vi "Acquisition Message Loop.vi"(6 "List Notifier":refnum<notifier>, 8 "error in (no error)":errorcluster, 9 "Data Queue":refnum<queue>, 10 "Data Notifier":refnum<notifier>, 11 "Message Queues":T1) -> (0 "error out":errorcluster)   [LabVIEW 2022 SP3, in "Acquisition.lvlib"]
doc: "Message loop for handling messages pertaining to the acquisition of data from the hardware."
uses:
  Acquisition.lvlib
  support/Message Queue/All Message Queues.ctl
  support/Message Queue/Message Cluster.ctl
  Hardware Configuration.ctl
  Acquisition State.ctl
  support/Message Queue/Enqueue Message (Single).vi
  <vilib>/Utility/error.llb/Error Cluster From Error Code.vi
  <vilib>/ErrorRing/Error Ring.xnode
  support/Message Queue/Message Queue.lvlib
  <instrlib>/BK Precision 911X Series/BK Precision 911X Series.lvlib
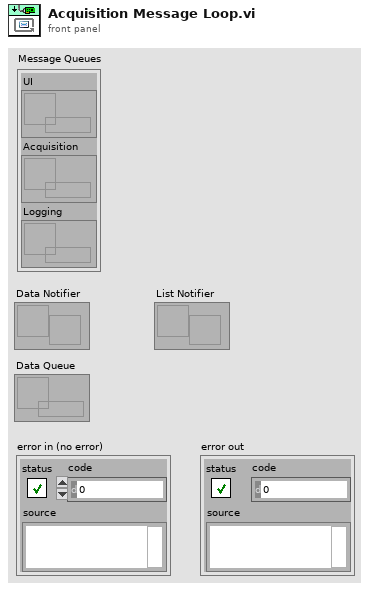
[diagram p1: front panel]
types:
  T1 = typedef "Message Queue.lvlib/All Message Queues.ctl" = cluster{"UI":refnum<queue>, "Acquisition":refnum<queue>, "Logging":refnum<queue>}
  T2 = typedef "Acquisition.lvlib/Hardware Configuration.ctl" = cluster{"VISA resource name":refnum<visa-resource-name>, "Baud Rate":u32, "Reset on Connect":bool, "Log Interval (s)":dbl, "Voltage":refnum<vi>, "Current":refnum<vi>, "Output Control":refnum<vi>}
  T3 = typedef "Acquisition.lvlib/Acquisition State.ctl" = enum16{"Idle", "Acquiring"}
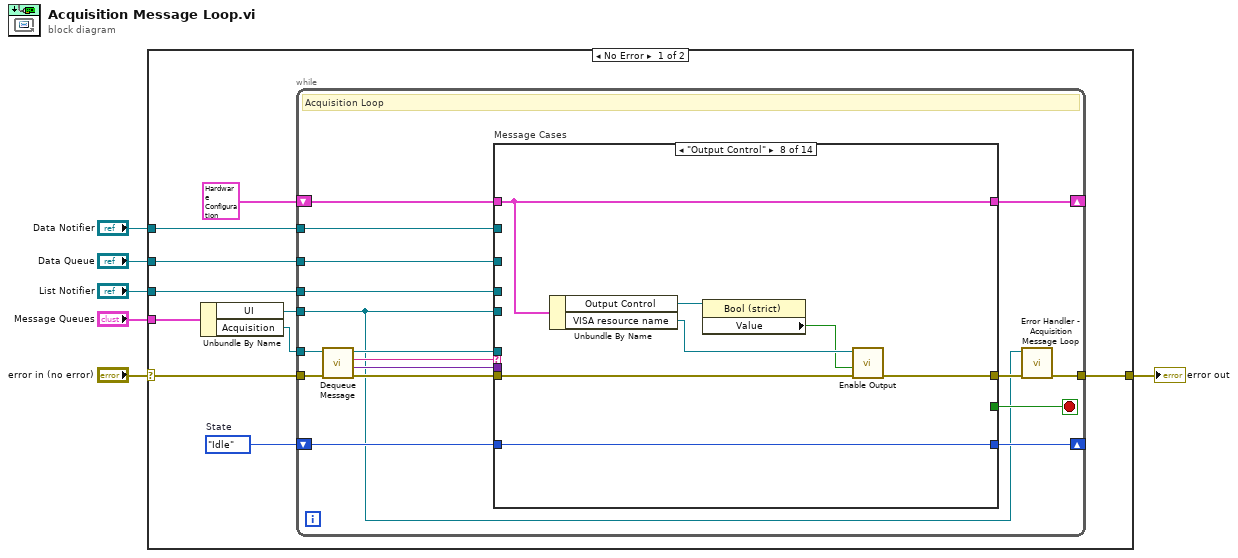
[diagram p0: block diagram]
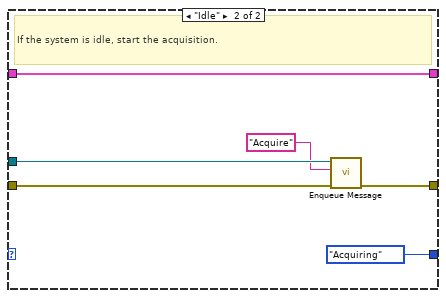
[diagram p4: hidden frame]
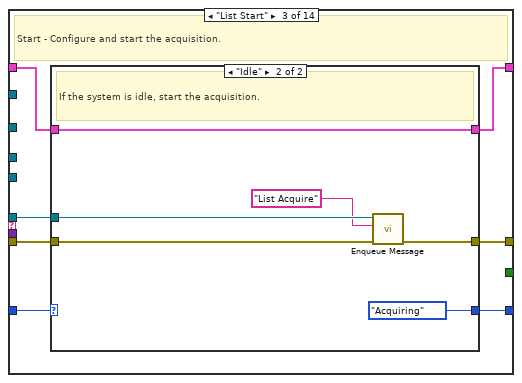
[diagram p5: hidden frame]
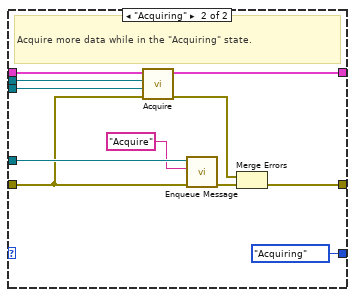
[diagram p8: hidden frame]
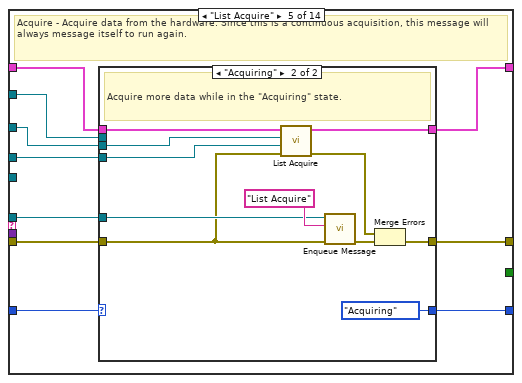
[diagram p9: hidden frame]
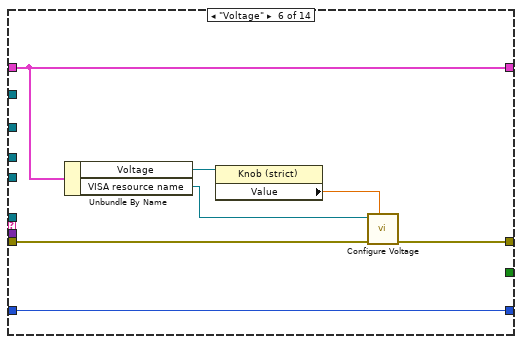
[diagram p11: hidden frame]
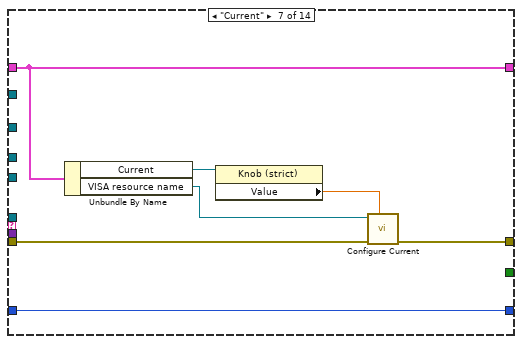
[diagram p12: hidden frame]
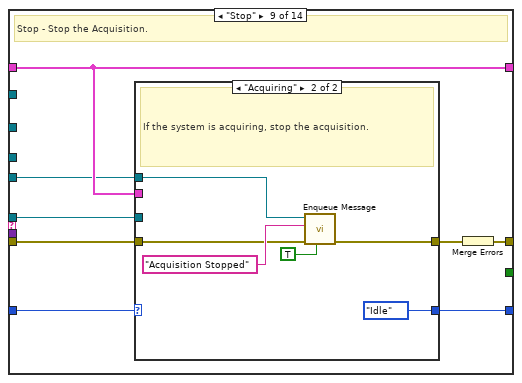
[diagram p13: hidden frame]
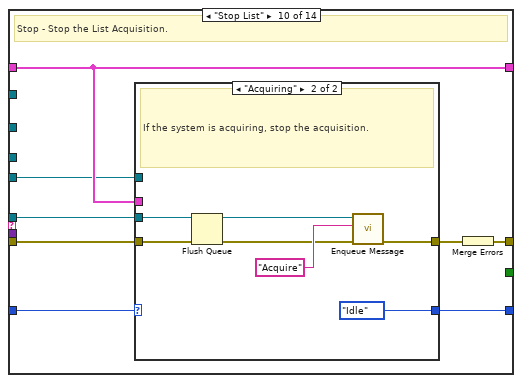
[diagram p15: hidden frame]
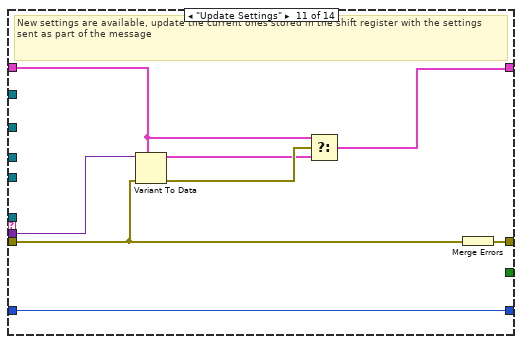
[diagram p17: hidden frame]
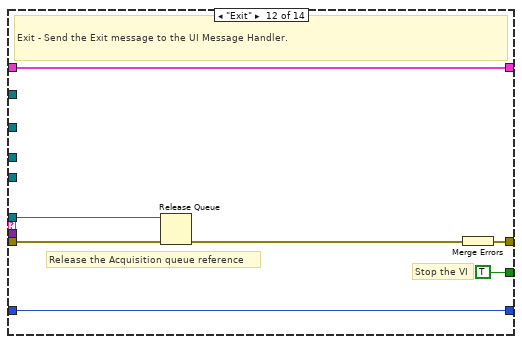
[diagram p18: hidden frame]
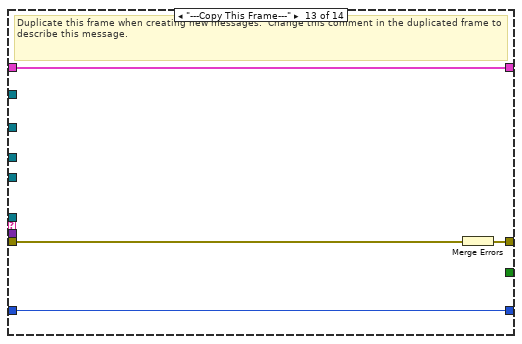
[diagram p19: hidden frame]
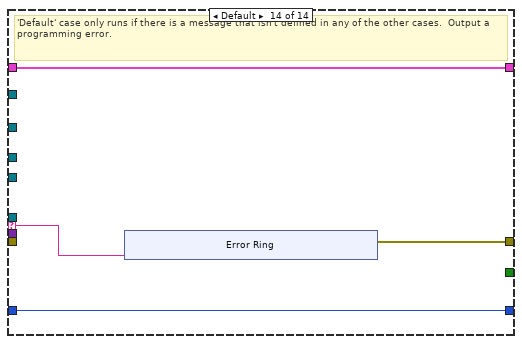
[diagram p20: hidden frame]
diagram:
  n1 = case shown="No Error" "error in (no error)" {
    selector: "error in (no error)" -> [w12 w200]
    tunnel: "Message Queues" -> [w16 _]
    tunnel: [w14 w200] -> w5
    tunnel: "Data Notifier" -> [w10 _]
    tunnel: "Data Queue" -> [w9 _]
    tunnel: "List Notifier" -> [w7 _]
    frame No Error {
      w8 = Acquisition_State."Idle"  # State
      n2 = Unbundle By Name(w16) -> ("UI"=w11:refnum<queue>, "Acquisition"=w15:refnum<queue>)
      n3 = while {
        tunnel: w15 -> [w26]
        shift-right: [w32] -> _
        shift-left: T2 {"VISA resource name"="", "Baud Rate"=0, "Reset on Connect"=FALSE, "Log Interval (s)"=0.0, "Voltage"=refnum, "Current"=refnum, "Output Control"=refnum} ("Data Cluster") -> [w33]
        tunnel: w11 -> [w18]
        tunnel: w10 -> [w25]
        tunnel: w9 -> [w24]
        shift-right: [w22] -> _
        shift-left: w8 -> [w23]
        tunnel: w12 -> [w30]
        tunnel: [w21] -> w14
        tunnel: w7 -> [w17]
        stop <- w31 stop-if-true
        # "Acquisition Loop"
        n4 = call "Dequeue Message.vi"("error in (no error)"=w30, "Message Queue"=w26) -> ("error out"=w29:errorcluster, "Message Data"=w27:variant, "Message"=w28:string, "dup Message Queue"=w19:refnum<queue>)  [unwired: 6 in]
        n5 = case "Message Cases" shown="\"Output Control\"" w28 {
          selector: w28 -> [_ _ _ _ _ _ _ _ _ _ _ _ _ w189]
          tunnel: w19 -> [_ w40 w56 w76 w100 _ _ _ w137 w153 _ w179 _ _]
          tunnel: w29 -> [w36 w41 w57 w75 w99 w121 w128 w135 w143 w159 w171 w181 w188 _]
          tunnel: [w36 w43 w59 w77 w101 w120 w127 w134 w144 w160 w177 w183 w186 w190] -> w20
          tunnel: w33 -> [w35 w42 w58 w73 w97 w119 w126 w133 w141 w157 w173 w182 w187 w192]
          tunnel: [w35 w39 w55 w74 w98 w119 w126 w133 w141 w157 w172 w182 w187 w192] -> w32
          tunnel: [_ _ _ _ _ _ _ _ _ _ _ TRUE _ _] -> w31
          tunnel: w27 -> [_ _ _ _ _ _ _ _ _ _ w176 _ _ _]
          tunnel: w18 -> [_ _ _ _ _ _ _ _ w138 w154 _ _ _ _]
          tunnel: w25 -> [_ _ _ w72 w96 _ _ _ _ _ _ _ _ _]
          tunnel: w24 -> [_ _ _ w71 w95 _ _ _ _ _ _ _ _ _]
          tunnel: w23 -> [w34 w37 w53 w69 w93 w122 w129 w136 w140 w156 w170 w178 w185 w191]
          tunnel: [w34 w38 w54 w70 w94 w122 w129 w136 w139 w155 w170 w178 w185 w191] -> w22
          tunnel: w17 -> [_ _ _ _ w92 _ _ _ _ _ _ _ _ _]
          frame "Initialize" {
            # "Initialize  - Initialize is currently a no-op.  The hardware initialization takes place in the 'Start' message."
          }
          frame "Start" {
            # "Start - Configure and start the acquisition."
            n6 = case shown="\"Acquiring\"" w37 {
              selector: w37 -> [w44 _]
              tunnel: [w45 w47] -> w43
              tunnel: w42 -> [w46 w52]
              tunnel: w41 -> [w45 w51]
              tunnel: w40 -> [_ w50]
              tunnel: [w46 w52] -> w39
              tunnel: [w44 Acquisition_State."Acquiring" ("Acquisition State")] -> w38
              frame "Acquiring" {
                # "The system is already acquiring. Ignore the \"Start\" message."
              }
              frame "Idle" {
                # "If the system is idle, start the acquisition."
                n7 = call-poly "Enqueue Message.vi"("error in (no error)"=w51, "Message"="Acquire", "Message Queue"=w50) -> ("error out"=w47:errorcluster)  [unwired: 7 in, 1 out]
              }
            }
          }
          frame "List Start" {
            # "Start - Configure and start the acquisition."
            n8 = case shown="\"Idle\"" w53 {
              selector: w53 -> [w60 _]
              tunnel: [w61 w63] -> w59
              tunnel: w58 -> [w62 w68]
              tunnel: w57 -> [w61 w67]
              tunnel: w56 -> [_ w66]
              tunnel: [w62 w68] -> w55
              tunnel: [w60 Acquisition_State."Acquiring" ("Acquisition State")] -> w54
              frame "Acquiring" {
                # "The system is already acquiring. Ignore the \"Start\" message."
              }
              frame "Idle" {
                # "If the system is idle, start the acquisition."
                n9 = call-poly "Enqueue Message.vi"("error in (no error)"=w67, "Message"="List Acquire", "Message Queue"=w66) -> ("error out"=w63:errorcluster)  [unwired: 7 in, 1 out]
              }
            }
          }
          frame "Acquire" {
            # "Acquire - Acquire data from the hardware. Since this is a continuous acquisition, this message will always message itself to run again."
            n10 = case shown="\"Idle\"" w69 {
              selector: w69 -> [w78 _]
              tunnel: [w79 w91] -> w77
              tunnel: w76 -> [_ w89]
              tunnel: w75 -> [w79 w82]
              tunnel: [w80 w87] -> w74
              tunnel: w73 -> [w80 w86]
              tunnel: w72 -> [_ w84]
              tunnel: w71 -> [_ w83]
              tunnel: [w78 Acquisition_State."Acquiring" ("State")] -> w70
              frame "Idle" {
                # "Ignore \"Acquire\" messages when the acquisition is idle."
              }
              frame "Acquiring" {
                # "Acquire more data while in the \"Acquiring\" state."
                n11 = call "Acquire.vi"("error in (no error)"=w82, "Data Queue"=w83, "Data Notifier"=w84, "Hardware Resources in"=w86) -> ("error out"=w88:errorcluster, "Hardware Resources out"=w87:T2)  [unwired: 6 in]
                n12 = call-poly "Enqueue Message.vi"("error in (no error)"=w82, "Message"="Acquire", "Message Queue"=w89) -> ("error out"=w90:errorcluster)  [unwired: 7 in, 1 out]
                n13 = Merge Errors(w88, w90) -> (w91:errorcluster)
              }
            }
          }
          frame "List Acquire" {
            # "Acquire - Acquire data from the hardware. Since this is a continuous acquisition, this message will always message itself to run again."
            n14 = case shown="\"Acquiring\"" w93 {
              selector: w93 -> [w102 _]
              tunnel: [w103 w115] -> w101
              tunnel: w100 -> [_ w106]
              tunnel: w99 -> [w103 w105]
              tunnel: [w104 w112] -> w98
              tunnel: w97 -> [w104 w111]
              tunnel: w96 -> [_ _]
              tunnel: w95 -> [_ w108]
              tunnel: [w102 Acquisition_State."Acquiring" ("State")] -> w94
              tunnel: w92 -> [_ w109]
              frame "Idle" {
                # "Ignore \"Acquire\" messages when the acquisition is idle."
              }
              frame "Acquiring" {
                # "Acquire more data while in the \"Acquiring\" state."
                n15 = call "List Acquire.vi"("error in (no error)"=w105, "List Notifier"=w109, "Data Queue"=w108, "Hardware Resources in"=w111) -> ("error out"=w113:errorcluster, "Hardware Resources out"=w112:T2)  [unwired: 6 in]
                n16 = call-poly "Enqueue Message.vi"("error in (no error)"=w105, "Message"="List Acquire", "Message Queue"=w106) -> ("error out"=w114:errorcluster)  [unwired: 7 in, 1 out]
                n17 = Merge Errors(w113, w114) -> (w115:errorcluster)
              }
            }
          }
          frame "Voltage" {
            n18 = Unbundle By Name(w119) -> ("Voltage"=w118:refnum<vi>, "VISA resource name"=w116:refnum<visa-resource-name>)
            n19 = property on="Property Node" class="Knob (strict)"(reference=w118) -> ("Value"=w117:dbl)  [unwired: 1 in, 2 out]
            n20 = call "Configure Voltage.vi"("Voltage"=w117, "error in (no error)"=w121, "VISA resource name"=w116) -> ("error out"=w120:errorcluster)  [unwired: 7 in, 1 out]
          }
          frame "Current" {
            n21 = Unbundle By Name(w126) -> ("Current"=w125:refnum<vi>, "VISA resource name"=w123:refnum<visa-resource-name>)
            n22 = property on="Property Node" class="Knob (strict)"(reference=w125) -> ("Value"=w124:dbl)  [unwired: 1 in, 2 out]
            n23 = call "Configure Current.vi"("Current"=w124, "error in (no error)"=w128, "VISA resource name"=w123) -> ("error out"=w127:errorcluster)  [unwired: 7 in, 1 out]
          }
          frame "Output Control" {
            n24 = Unbundle By Name(w133) -> ("Output Control"=w132:refnum<vi>, "VISA resource name"=w131:refnum<visa-resource-name>)
            n25 = property on="Property Node" class="Bool (strict)"(reference=w132) -> ("Value"=w130:bool)  [unwired: 1 in, 2 out]
            n26 = call <instrlib>:"Enable Output.vi"("error in (no error)"=w135, "Enable Output (F: False)"=w130, "VISA resource name"=w131) -> ("error out"=w134:errorcluster)  [unwired: 7 in, 1 out]
          }
          frame "Stop" {
            # "Stop - Stop the Acquisition."
            n27 = case shown="\"Acquiring\"" w140 {
              selector: w140 -> [w145 _]
              tunnel: w143 -> [w146 w147]
              tunnel: [w146 w149] -> w142
              tunnel: w141 -> [_ _]
              tunnel: [w145 Acquisition_State."Idle" ("State")] -> w139
              tunnel: w138 -> [_ w151]
              tunnel: w137 -> [_ _]
              frame "Idle" {
                # "The system is already idle. Ignore the \"Stop\" message."
              }
              frame "Acquiring" {
                # "If the system is acquiring, stop the acquisition."
                n28 = call-poly "Enqueue Message.vi"("Priority Message? (F)"=TRUE, "error in (no error)"=w147, "Message"="Acquisition Stopped", "Message Queue"=w151) -> ("error out"=w149:errorcluster)  [unwired: 6 in, 1 out]
              }
            }
            n29 = Merge Errors(w142) -> (w144:errorcluster)
          }
          frame "Stop List" {
            # "Stop - Stop the List Acquisition."
            n30 = case shown="\"Acquiring\"" w156 {
              selector: w156 -> [w161 _]
              tunnel: w159 -> [w162 w166]
              tunnel: [w162 w168] -> w158
              tunnel: w157 -> [_ _]
              tunnel: [w161 Acquisition_State."Idle" ("State")] -> w155
              tunnel: w154 -> [_ _]
              tunnel: w153 -> [_ w164]
              frame "Idle" {
                # "The system is already idle. Ignore the \"Stop\" message."
              }
              frame "Acquiring" {
                # "If the system is acquiring, stop the acquisition."
                n31 = Flush Queue(queue=w164, error in (no error)=w166) -> (queue out=w163:refnum<queue>, error out=w165:errorcluster)  [unwired: 1 out]
                n32 = call-poly "Enqueue Message.vi"("error in (no error)"=w165, "Message"="Acquire", "Message Queue"=w163) -> ("error out"=w168:errorcluster)  [unwired: 7 in, 1 out]
              }
            }
            n33 = Merge Errors(w158) -> (w160:errorcluster)
          }
          frame "Update Settings" {
            # "New settings are available, update the current ones stored in the shift register with the settings sent as part of the message"
            n34 = Variant To Data(error in=w171, type=w173, Variant=w176) -> (data=w174:T2, error out=w175:errorcluster)
            n35 = Select(t=w173, s=w175, f=w174) -> (s? t:f=w172:T2)
            n36 = Merge Errors(w171) -> (w177:errorcluster)
          }
          frame "Exit" {
            # "Release the Acquisition queue reference"
            # "Stop the VI"
            # "Exit - Send the Exit message to the UI Message Handler."
            n37 = Release Queue(queue=w179, error in (no error)=w181) -> (error out=w180:errorcluster)  [unwired: 1 in, 2 out]
            n38 = Merge Errors(w180) -> (w183:errorcluster)
          }
          frame "---Copy This Frame---" {
            # "Duplicate this frame when creating new messages.  Change this comment in the duplicated frame to describe this message."
            n39 = Merge Errors(w188) -> (w186:errorcluster)
          }
          frame Default {
            # "'Default' case only runs if there is a message that isn't defined in any of the other cases.  Output a programming error."
            n40 = xnode "Error Ring"("parameter 0"=w189) -> ("error out"=w190:errorcluster)
          }
        }
        n41 = call "Error Handler - Acquisition Message Loop.vi"("error in (no error)"=w20, "Message Queue"=w18) -> ("dup error in"=w21:errorcluster)  [unwired: 8 in, 1 out]
      }
    }
    frame Error {
    }
  }
  "error out" <- w5
